vi "Untitled 9.vi"() -> ()   [LabVIEW 2014, in "Files Library.lvlib"]
uses:
  Files Library.lvlib
  <vilib>/NI/Modbus Library/API/Master/Modbus Master.lvclass
panel:
  out "Current Time 2":u16[](array[numeric])
  in  "Time Setpoint 2":u16
  in  "C1 2":bool
  in  "C3 2":bool
  out "Array":u16[](array[numeric])
  in  "Right":bool
  in  "Left":bool
  in  "Modbus master in":refnum<class "Modbus Master.lvclass">
  in  "error in":errorcluster
  in  "Start":bool
  in  "stop":bool
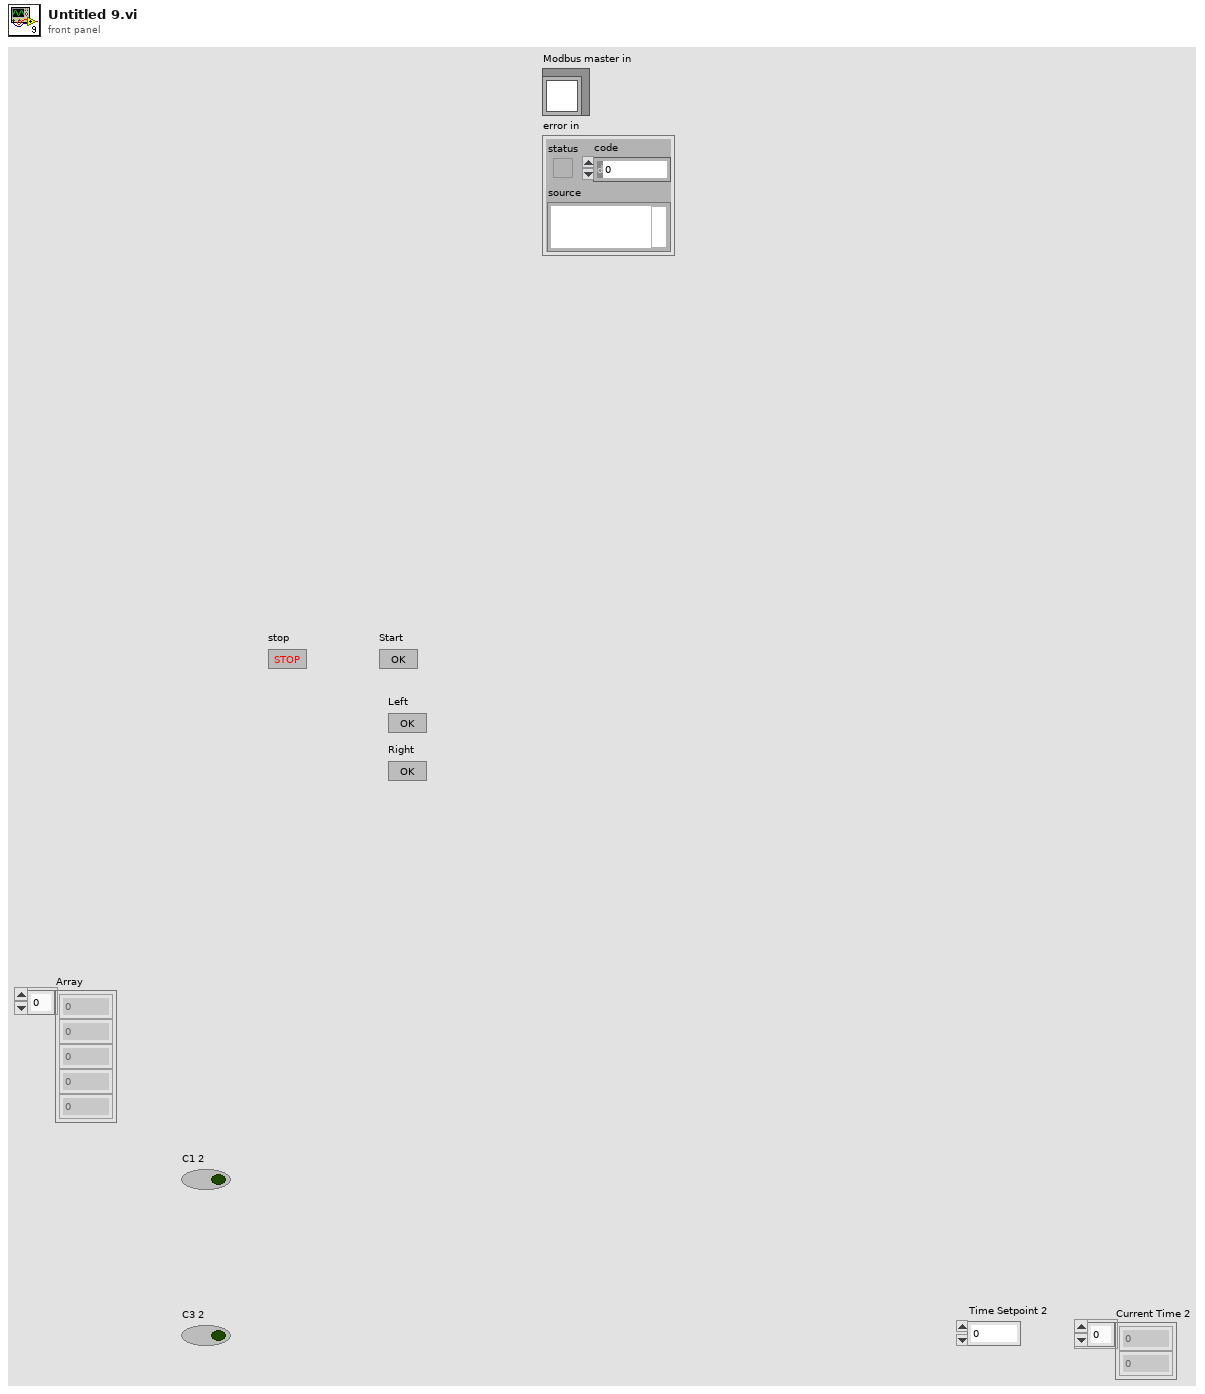
[diagram p1: front panel]
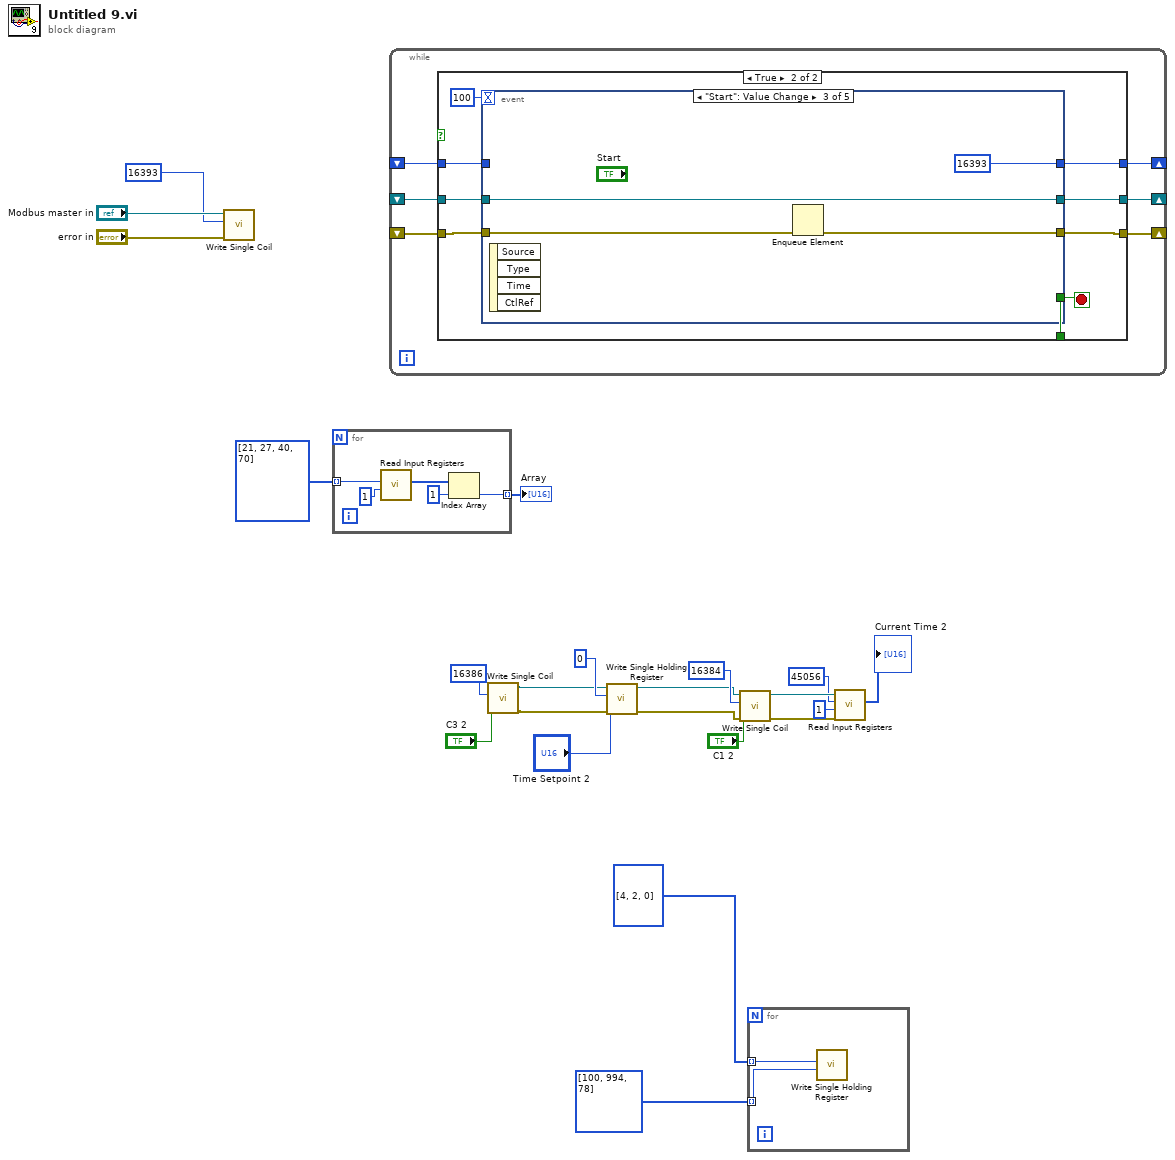
[diagram p0: block diagram]
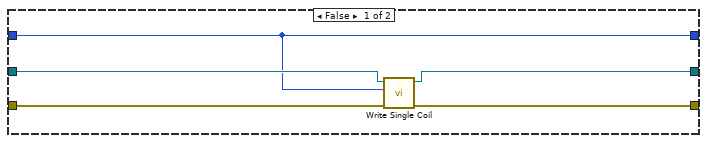
[diagram p2: hidden frame]
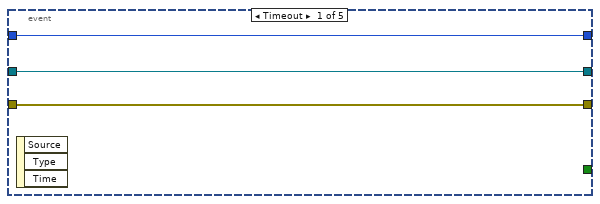
[diagram p3: hidden frame]
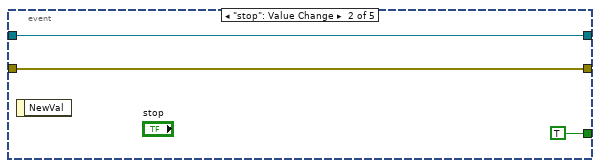
[diagram p4: hidden frame]
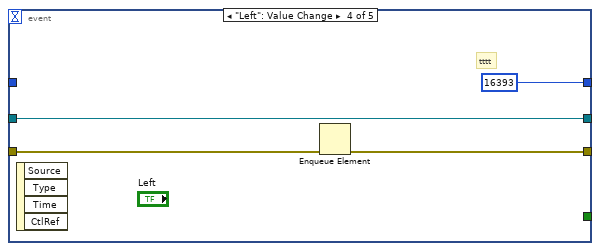
[diagram p5: hidden frame]
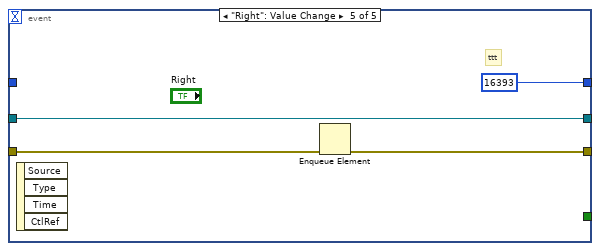
[diagram p6: hidden frame]
diagram:
  n1 = call-dynamic "Write Single Coil.vi"("error in"="error in", "address"=u16 16393, "Modbus master in"="Modbus master in") -> ("coil to write"=w25:bool)  [unwired: 6 in, 2 out]
  n2 = for {
    tunnel: u16[] [21, 27, 40, 70] -> [w30] mode=indexing
    tunnel: [w26] -> w20 mode=indexing
    n3 = call-dynamic "Read Input Registers.vi"("number of inputs"=u16 1, "starting address"=w30) -> ("register values"=w28:u16[])  [unwired: 7 in, 2 out]
    n4 = Index Array(array=w28, index=1) -> (element=w26:u16)
  }
  "Array" <- w20
  n5 = while {
    shift-right: [w35] -> _
    shift-left: _ -> [w36]
    shift-right: [w34] -> _
    shift-left: _ -> [w33]
    shift-right: [w32] -> _
    shift-left: _ -> [w31]
    stop <- w37 stop-if-true
    n6 = case shown="True" {
      selector: _ -> [_ _]
      tunnel: [_ w49] -> w37
      tunnel: w36 -> [w42 w47]
      tunnel: [w41 w48] -> w35
      tunnel: [w40 w46] -> w34
      tunnel: w33 -> [w39 w45]
      tunnel: [w38 w44] -> w32
      tunnel: w31 -> [w38 w43]
      frame False {
        n7 = call-dynamic "Write Single Coil.vi"("error in"=w42, "address"=w38, "Modbus master in"=w39) -> ("error out"=w41:errorcluster, "Modbus master out"=w40:refnum<class "Modbus Master.lvclass">)  [unwired: 7 in]
      }
      frame True {
        n8 = event shown="[2] \"Start\": Value Change" {
          selector: _ -> [_ _ _ _ _]
          dyn-events: _ -> [_ _ _ _ _]
          timeout: 100 -> [_ _ _ _ _]
          tunnel: [_ TRUE _ _ _] -> w49
          tunnel: [w51 w54 w57 w61 w65] -> w48
          tunnel: w47 -> [w51 w54 w58 w62 w66]
          tunnel: [w52 w55 w60 w64 w68] -> w46
          tunnel: w45 -> [w52 w55 w60 w64 w68]
          tunnel: [w53 _ u16 16393 ("address") u16 16393 ("address") u16 16393 ("address")] -> w44
          tunnel: w43 -> [w53 _ _ _ _]
          event Timeout {
            n9 = event-data() -> ()  [unwired: 1 in, 3 out]
          }
          event "stop": Value Change {
            n10 = event-data() -> ()  [unwired: 1 in, 1 out]
          }
          event "Start": Value Change {
            n11 = event-data() -> ()  [unwired: 1 in, 4 out]
            n12 = Enqueue Element(error in (no error)=w58) -> (error out=w57:errorcluster)  [unwired: 3 in, 2 out]
          }
          event "Left": Value Change {
            # "tttt"
            n13 = event-data() -> ()  [unwired: 1 in, 4 out]
            n14 = Enqueue Element(error in (no error)=w62) -> (error out=w61:errorcluster)  [unwired: 3 in, 2 out]
          }
          event "Right": Value Change {
            # "ttt"
            n15 = event-data() -> ()  [unwired: 1 in, 4 out]
            n16 = Enqueue Element(error in (no error)=w66) -> (error out=w65:errorcluster)  [unwired: 3 in, 2 out]
          }
        }
      }
    }
  }
  n17 = call-dynamic "Write Single Coil.vi"("coil to write"="C3 2", "address"=u16 16386) -> ("error out"=w10:errorcluster, "Modbus master out"=w11:refnum<class "Modbus Master.lvclass">)  [unwired: 8 in]
  n18 = call-dynamic "Write Single Holding Register.vi"("error in"=w10, "register to write"="Time Setpoint 2", "address"=u16 0, "Modbus master in"=w11) -> ("error out"=w13:errorcluster, "Modbus master out"=w12:refnum<class "Modbus Master.lvclass">)  [unwired: 6 in]
  n19 = call-dynamic "Write Single Coil.vi"("error in"=w13, "coil to write"="C1 2", "address"=u16 16384, "Modbus master in"=w12) -> ("error out"=w8:errorcluster, "Modbus master out"=w9:refnum<class "Modbus Master.lvclass">)  [unwired: 6 in]
  n20 = for {
    tunnel: u16[] [4, 2, 0] -> [w70] mode=indexing
    tunnel: u16[] [100, 994, 78] -> [w69] mode=indexing
    n21 = call-dynamic "Write Single Holding Register.vi"("register to write"=w69, "address"=w70) -> ()  [unwired: 8 in, 2 out]
  }
  n22 = call-dynamic "Read Input Registers.vi"("error in"=w8, "number of inputs"=u16 1, "starting address"=u16 45056, "Modbus master in"=w9) -> ("error out"=w3:errorcluster, "register values"=→"Current Time 2":u16[], "Modbus master out"=w4:refnum<class "Modbus Master.lvclass">)  [unwired: 5 in]
